vi "ID_List.vi"() -> ()   [LabVIEW 2024]
panel:
  out "ID_list":u16[](array[numeric])
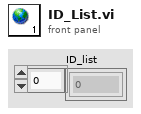
[diagram p1: front panel]
diagram:
